vi "onAddVerboseExplanation.vi"(5 "append":bool, 7 "overwrite":bool, 8 "error in (no error)":errorcluster, 10 "Verbose Explanation":string, 11 "Leaf in":refnum<class "Leaf.lvclass">) -> (0 "error out":errorcluster, 3 "Leaf out":refnum<class "Leaf.lvclass">)   [LabVIEW 2021, in "Bananas.lvlib" / "Leaf.lvclass"]
uses:
  Leaf.lvclass
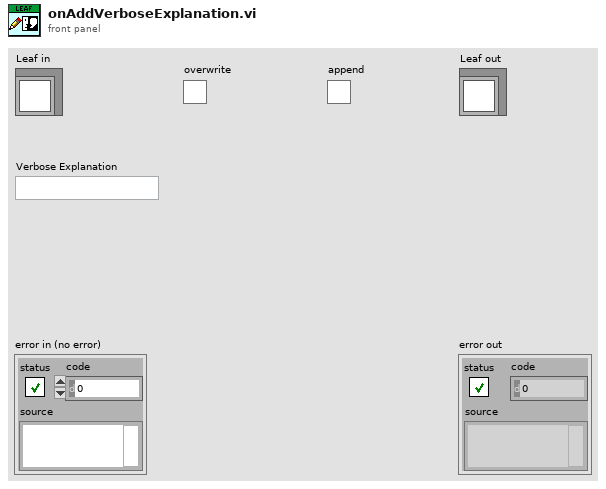
[diagram p1: front panel]
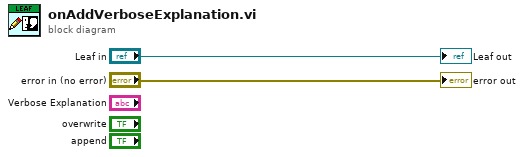
[diagram p0: block diagram]
diagram:
  "error out" <- "error in (no error)"
  "Leaf out" <- "Leaf in"
